vi "set_scale_bar_state.vi"(8 "error in (no error)":errorcluster, 10 "enable?":bool, 11 "Image in":refnum<class "Image.lvclass">) -> (0 "error out":errorcluster, 3 "Image out":refnum<class "Image.lvclass">)   [LabVIEW 2010, in "Image.lvclass"]
uses:
  Image.lvclass
  Image.lvclass/Image.ctl
  <vilib>/vision/Image Controls.llb/IMAQ Image.ctl
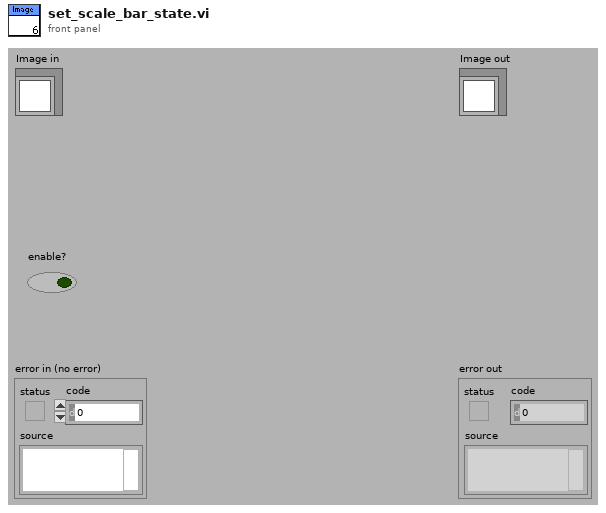
[diagram p1: front panel]
types:
  T1 = typedef "IMAQ Image.ctl" = refnum<image>
  T2 = typedef "Image.lvclass/storage_mode.ctl" = enum16{"RAM", "disk"}
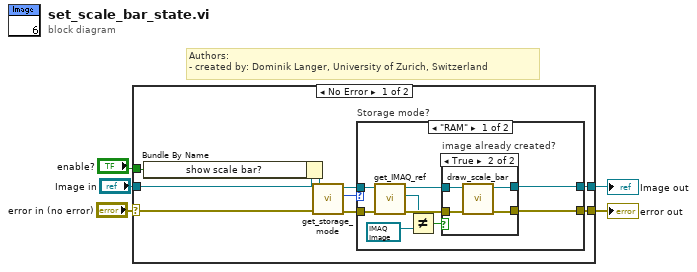
[diagram p0: block diagram]
diagram:
  # "Authors: \n- created by: Dominik Langer, University of Zurich, Switzerland"
  n1 = case shown="No Error" "error in (no error)" {
    selector: "error in (no error)" -> [w8 w33]
    tunnel: [w11 w33] -> w4
    tunnel: [w12 w32] -> w2
    tunnel: "Image in" -> [w14 w32]
    tunnel: "enable?" -> [w13 _]
    frame No Error {
      n2 = Bundle By Name(cluster=w14, "show scale bar?"=w13) -> (w10:refnum<class "Image.lvclass">)
      n3 = call-dynamic "get_storage_mode.vi"("error in (no error)"=w8, "Image.lvclass in"=w10) -> ("error out"=w7:errorcluster, "storage mode"=w6:T2, "Image.lvclass out"=w9:refnum<class "Image.lvclass">)  [unwired: 7 out]
      n4 = case "Storage mode?" shown="\"RAM\"" w6 {
        tunnel: [w23 w31] -> w12
        tunnel: [w22 w30] -> w11
        tunnel: w9 -> [w19 w31]
        tunnel: w7 -> [w21 w30]
        frame "RAM" {
          n5 = call-dynamic "get_IMAQ_ref.vi"("error in (no error)"=w21, "Image.lvclass in"=w19) -> ("error out"=w20:errorcluster, "Image"=w16:T1, "Image.lvclass out"=w18:refnum<class "Image.lvclass">)  [unwired: 7 out]
          n6 = Not Equal?(x=w16, y=T1 refnum ("Image")) -> (x != y?=w17:bool)
          n7 = case "image already created?" shown="True" w17 {
            tunnel: [w25 w29] -> w23
            tunnel: [w24 w28] -> w22
            tunnel: w20 -> [w24 w27]
            tunnel: w18 -> [w25 w26]
            frame False {
            }
            frame True {
              n8 = call "draw_scale_bar.vi"("error in (no error)"=w27, "Image in"=w26) -> ("error out"=w28:errorcluster, "Image out"=w29:refnum<class "Image.lvclass">)  [unwired: 3 in, 5 out]
            }
          }
        }
        frame "disk", Default {
        }
      }
    }
    frame Error {
    }
  }
  "error out" <- w4
  "Image out" <- w2
